vi "Rows to Ch_names.vi"(1 "array type (2D Dbl)":string[][](array[string])) -> (0 "Array":string[](array[string]))   [LabVIEW 2016]
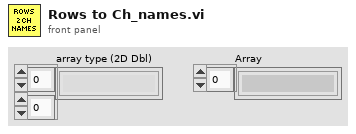
[diagram p1: front panel]
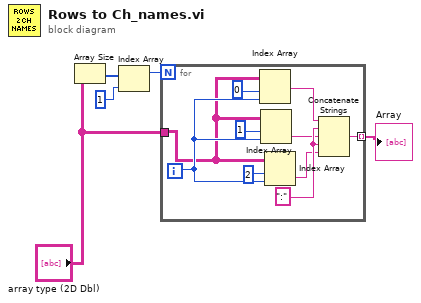
[diagram p0: block diagram]
diagram:
  n1 = Array Size(array="array type (2D Dbl)") -> (size(s)=w1:i32[])
  n2 = Index Array(array=w1, index=1 ("Index")) -> (element=w4:i32)
  n3 = for {
    N: w4 -> [_]
    tunnel: "array type (2D Dbl)" -> [w10]
    tunnel: [w6] -> w5 mode=indexing
    i -> [w14]
    w15 = ":"
    n4 = Index Array(array=w10, index (row)=0 ("Index"), index (col)=w14) -> (element=w9:string)
    n5 = Index Array(array=w10, index (row)=1 ("Index"), index (col)=w14) -> (element=w8:string)
    n6 = Index Array(array=w10, index (row)=2 ("Index"), index (col)=w14) -> (element=w7:string)
    n7 = Concatenate Strings(w9, w15, w8, w15, w7) -> (w6:string)
  }
  "Array" <- w5
